vi "Pfeiffer Vacuum Turbo Config A D input output.vi"(8 "error in (no error)":errorcluster, 9 "PV config A D input output - Cluster":T1={"Parameter"=enum." Configuration DO2 (019)", "Parameter\nread only<->describe"=FALSE, "off<->on   "=TRUE, "Configuration DO1 / DO2 / R1 / R2 / R3"=0, "Configuration AO1"=0, "Config. Acces. A1/A2"=0, "Config. Acces. B1/B2"=0, "Configuration DI1 / DI2 / DI3"=0} {"Configuration DI1 / DI2 / DI3" items=[" speed", " power", " current", " lowest value", " highest value"]; "Config. Acces. B1/B2" items=[" fan (constant) (default)", " venting valve", " heating", " backing pump", " fan (temperature controlled)", " seal gas", " always off", " always on"]; "Config. Acces. A1/A2" items=[" fan (constant)", " venting valve", " heating", " backing pump", " fan (temperature controlled)", " seal gas", " always off", " always on"]; "Configuration DO1 / DO2 / R1 / R2 / R3" items=[" switchpoint attained", " no error", " error", " warning", " error and/or warning", " set speed attained", " pump is on", " accelerates", " decelerater", " always off", " always on", " access request remote"]; "Configuration AO1" items=[" speed", " power", " current", " lowest value", " highest value"]}, 10 "Adress of unit":u16=1 min=1 max=999 step=1, 11 "COM Port Name in":refnum<visa-resource-name>="COM1") -> (0 "error out":errorcluster, 3 "response (data)":string)   [LabVIEW 2016]
doc: "This VI is an example of how to use the Pfeiffer Vacuum subVIs programmatically. This VI first initializes the instrument, takes measurements, then closes the instrument."
uses:
  Public/Turbopumps/PV config A D input output - Cluster.ctl
  Pfeiffer Vacuum.lvlib
panel:
  # "Configuration heating output K4    : \n Configuration AI 1                             :"
  # "<--------------\n  false\n  heat/TMS\n  disabled"
  # "----------->          \ntrue \nsealing gas valve control \n set speed"
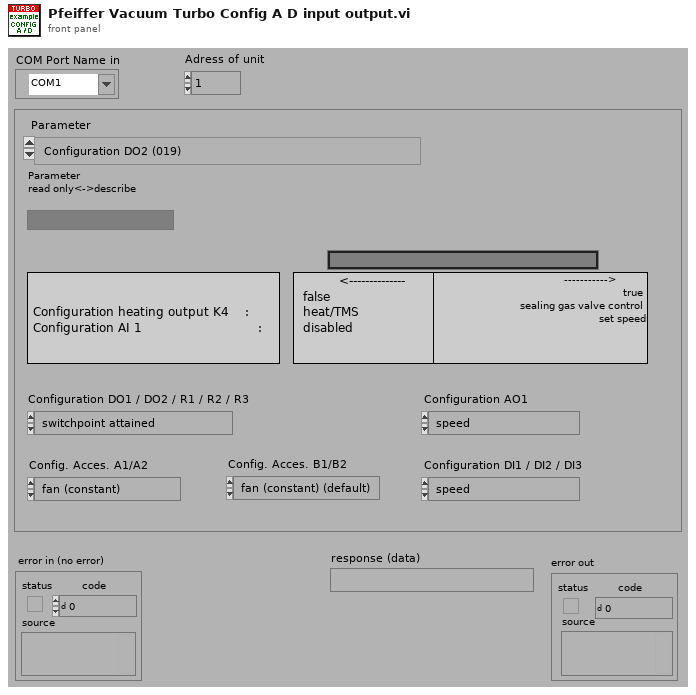
[diagram p1: front panel]
types:
  T1 = typedef "Pfeiffer Vacuum.lvlib/PV config A D input output - Cluster.ctl" = cluster{"Parameter":enum16{" Configuration DO2 (019)", " Configuration DO1 (024)", " Configuration heating output (032)", " Configuration accessory A1 (035)", " Configuration accessory B1 (036)", " Configuration accessory A2 (037)", " Configuration accessory B2 (038)", " Configuration Relais 1 (045)", " Configuration Relais 2 (046)", " Configuration Relais 3 (047)", " Configuration AO1 (055)", " Configuration AI1 (057)", " Configuration DI1 (062)", " Configuration DI2 (063)", " Configuration DI3 (064)"}, "Parameter\nread only<->describe":bool, "off<->on   ":bool, "Configuration DO1 / DO2 / R1 / R2 / R3":u16, "Configuration AO1":u16, "Config. Acces. A1/A2":u16, "Config. Acces. B1/B2":u16, "Configuration DI1 / DI2 / DI3":u16}
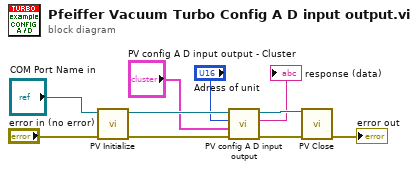
[diagram p0: block diagram]
diagram:
  n1 = call "PV Initialize.vi"("error in (no error)"="error in (no error)", "VISA session in"="COM Port Name in") -> ("error out"=w10:errorcluster, "VISA session out"=w8:refnum<visa-resource-name>)  [unwired: 8 in]
  n2 = call "PV config A D input output.vi"("error in (no error)"=w10, "PV config A D input output - Cluster"="PV config A D input output - Cluster", "Adress of unit"="Adress of unit", "VISA session"=w8) -> ("error out"=w9:errorcluster, "response (data)"=→"response (data)":string, "dup VISA session"=w7:refnum<visa-resource-name>)  [unwired: 5 in]
  n3 = call "PV Close.vi"("VISA session"=w7, "error in (no error)"=w9) -> ("error out"=→"error out":errorcluster)  [unwired: 13 in]
